vi "Initialize.vi"(7 "ChannelName":string="Setpoint.ch%d.SP", 8 "error in":errorcluster, 9 "Number of Channels":u32=1, 10 "Instance Name":string, 11 "Parallel Mode in":refnum<class "Parallel Mode.lvclass">) -> (0 "error out":errorcluster, 2 "Channel":T1[](array[typedef]), 3 "Parallel Mode out":refnum<class "Parallel Mode.lvclass">)   [LabVIEW 2023, in "Parallel Mode.lvclass"]
uses:
  Parallel Mode.lvclass
  Utilities/Channel.ctl
  Parallel Mode.lvclass/Parallel Mode.ctl
  <vilib>/ADAS Replay HIL/Channels/Tag Wrapper/Polymorphic/Open Consumer Tag (Boolean).vi
  <vilib>/ADAS Replay HIL/Channels/Tag Wrapper/Polymorphic/Set Default Value (Boolean).vi
  <vilib>/ADAS Replay HIL/Channels/Tag Wrapper/Polymorphic/Open Producer Tag (I32).vi
  <vilib>/ADAS Replay HIL/Channels/Tag Wrapper/Polymorphic/Set Default Value (I32).vi
  <vilib>/ADAS Replay HIL/Channels/Tag Wrapper/Polymorphic/Open Consumer Tag (Boolean).vi/bacb721e-673a-491a-accd-959f2e1f334e.vi
  <vilib>/ADAS Replay HIL/Channels/Tag Wrapper/Polymorphic/Set Default Value (Boolean).vi/228e99de-6fcf-414d-86fc-dc277c7b351f.vi
  <vilib>/ADAS Replay HIL/Channels/Tag Wrapper/Polymorphic/Open Producer Tag (I32).vi/45cd6eaa-a1ce-41a4-8aba-62a49d103d7e.vi
  <vilib>/ADAS Replay HIL/Channels/Tag Wrapper/Polymorphic/Set Default Value (I32).vi/228e99de-6fcf-414d-86fc-dc277c7b351f.vi
  <vilib>/ADAS Replay HIL/Channels/Tag Wrapper/Polymorphic/Open Consumer Tag (Boolean).vi/bacb721e-673a-491a-accd-959f2e1f334e.vi/c28b0ead-42ad-4072-80a2-aca7f2bd7ce3.vi
  <vilib>/ADAS Replay HIL/Channels/Tag Wrapper/Polymorphic/Set Default Value (Boolean).vi/228e99de-6fcf-414d-86fc-dc277c7b351f.vi/4bc1c15b-36ab-481f-b8dd-c64075ce723a.vi
  <vilib>/ADAS Replay HIL/Channels/Tag Wrapper/Polymorphic/Open Producer Tag (I32).vi/45cd6eaa-a1ce-41a4-8aba-62a49d103d7e.vi/c28b0ead-42ad-4072-80a2-aca7f2bd7ce3.vi
  <vilib>/ADAS Replay HIL/Channels/Tag Wrapper/Polymorphic/Set Default Value (I32).vi/228e99de-6fcf-414d-86fc-dc277c7b351f.vi/4bc1c15b-36ab-481f-b8dd-c64075ce723a.vi
  <vilib>/ADAS Replay HIL/AdasHilServices/AdasHilServices Fill In Error Info Ex.vi
  Utilities/Utilities.lvlib
  adas-replay-hil-internal/source/Channels/Tag Wrapper/Tag Wrapper.lvlib
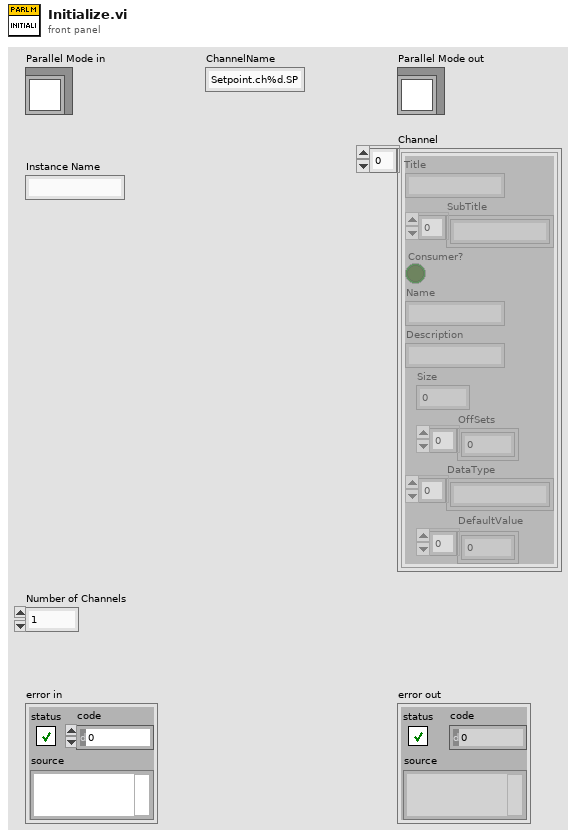
[diagram p1: front panel]
types:
  T1 = typedef "Utilities.lvlib/Channel.ctl" = cluster{"Title":string, "SubTitle":string[], "Consumer?":bool, "Name":string, "Description":string, "Size":i32, "OffSets":i32[], "DataType":string[], "DefaultValue":dbl[]}
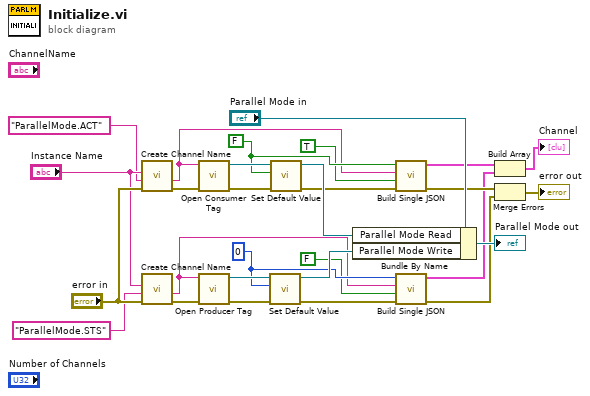
[diagram p0: block diagram]
diagram:
  w9 = 0 ("Default Value")
  w8 = FALSE ("Default Value")
  n1 = call "Create Channel Name.vi"("error in"="error in", "Channel Name"="ParallelMode.ACT", "Plugin Name"="Instance Name") -> ("error out"=w28:errorcluster, "Data Channel Name"=w7:string)  [unwired: 7 in]
  n2 = call "Create Channel Name.vi"("error in"="error in", "Channel Name"="ParallelMode.STS", "Plugin Name"="Instance Name") -> ("error out"=w22:errorcluster, "Data Channel Name"=w6:string)  [unwired: 7 in]
  n3 = call-poly <vilib>:"Open Consumer Tag.vi"("error in"=w28, "Channel Name"=w7) -> ("error out"=w27:errorcluster, "ADAS HIL Channel"=w26:refnum<k21>)  [unwired: 8 in]
  n4 = call-poly <vilib>:"Open Producer Tag.vi"("error in"=w22, "Channel Name"=w6) -> ("error out"=w21:errorcluster, "ADAS HIL Channel"=w23:refnum<k21>)  [unwired: 8 in]
  n5 = call-poly <vilib>:"Set Default Value.vi"("error in"=w21, "Default Value"=w9, "ADAS HIL Channel in"=w23) -> ("error out"=w11:errorcluster, "ADAS HIL Channel out"=w24:refnum<k21>)  [unwired: 7 in]
  n6 = call-poly <vilib>:"Set Default Value.vi"("error in"=w27, "Default Value"=w8, "ADAS HIL Channel in"=w26) -> ("error out"=w13:errorcluster, "ADAS HIL Channel out"=w25:refnum<k21>)  [unwired: 7 in]
  n7 = Bundle By Name(cluster="Parallel Mode in", "Parallel Mode Read"=w25, "Parallel Mode Write"=w24) -> (→"Parallel Mode out":refnum<class "Parallel Mode.lvclass">)
  n8 = call "Build Single JSON.vi"("error in"=w13, "Consumer?"=TRUE, "ChannelName"=w7, "Single"=w8) -> ("error out"=w12:errorcluster, "Channel"=w2:T1)  [unwired: 6 in]
  n9 = call "Build Single JSON.vi"("error in"=w11, "Consumer?"=FALSE, "ChannelName"=w6, "Single"=w9) -> ("error out"=w10:errorcluster, "Channel"=w3:T1)  [unwired: 6 in]
  n10 = Build Array(w2, w3) -> (→"Channel":T1[])
  n11 = Merge Errors(w12, w10) -> (→"error out":errorcluster)
